vi "DemoClass1_Create.vi"(0 "reference in":refnum<class "DemoClass1.lvclass">, 5 "error in (no error)":errorcluster) -> (14 "reference out":refnum<class "DemoClass1.lvclass">, 19 "error out":errorcluster)   [LabVIEW 2020, in "DemoClass1.lvclass"]
uses:
  <vilib>/addons/GOOPUtility/_Demo/GOOPUtil_Demo/DemoClass1_class/DemoClass1.lvclass
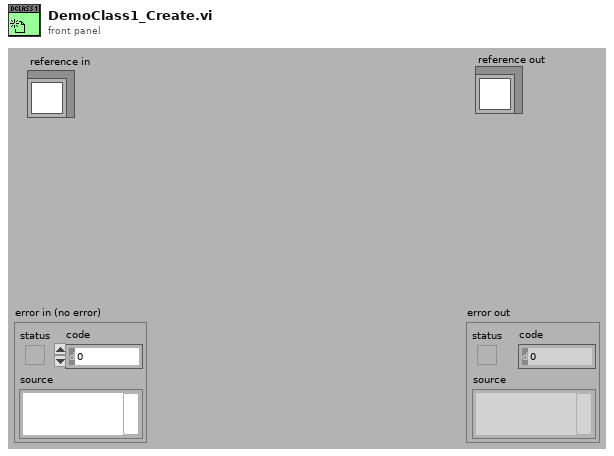
[diagram p1: front panel]
types:
  T1 = enum16{"Create", "Create or look up existing", "Look up existing"}
  T2 = typedef "DemoClass1.lvclass/ObjectAttributes.ctl" = cluster{"Attribute1":dbl}
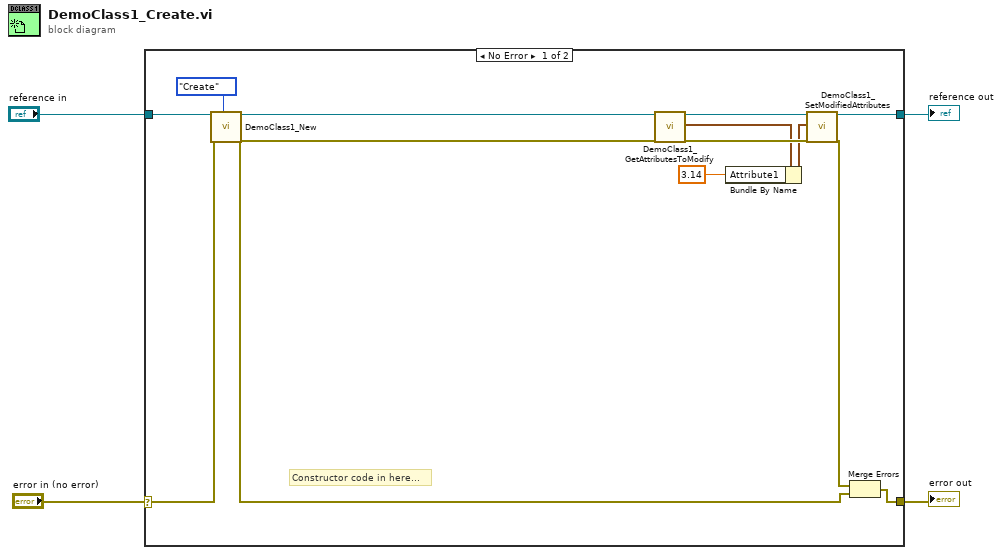
[diagram p0: block diagram]
diagram:
  n1 = case shown="No Error" "error in (no error)" {
    selector: "error in (no error)" -> [w17 w19]
    tunnel: [w8 w19] -> w4
    tunnel: "reference in" -> [w10 w18]
    tunnel: [w11 w18] -> w2
    frame No Error {
      # "Constructor code in here..."
      n2 = call <vilib>:"DemoClass1_New.vi"("reference in"=w10, "error in (no error)"=w17, "Create method"=T1."Create") -> ("reference out"=w9:refnum<class "DemoClass1.lvclass">, "error out"=w6:errorcluster)  [unwired: 13 in, 2 out]
      n3 = call <vilib>:"DemoClass1_GetAttributesToModify.vi"("reference in"=w9, "error in (no error)"=w6) -> ("reference out"=w15:refnum<class "DemoClass1.lvclass">, "Attributes"=w14:T2, "error out"=w16:errorcluster)  [unwired: 14 in, 1 out]
      n4 = Bundle By Name(cluster=w14, "Attribute1"=3.14 ("attribute1")) -> (w13:T2)
      n5 = call <vilib>:"DemoClass1_SetModifiedAttributes.vi"("reference in"=w15, "Attributes"=w13, "error in (no error)"=w16) -> ("reference out"=w11:refnum<class "DemoClass1.lvclass">, "error out"=w7:errorcluster)  [unwired: 15 in]
      n6 = Merge Errors(w7, w6) -> (w8:errorcluster)
    }
    frame Error {
    }
  }
  "error out" <- w4
  "reference out" <- w2
